vi "parse_channel_list.vi"(8 "error in (no error)":errorcluster, 11 "Channels Control":string[][](table)=[["camera", "1", "1", "", "", "", "", "", "", "", "", "", "", "", "", "", "", "", "", ""], ["probe", "1", "0", "", "", "", "", "", "", "", "", "", "", "", "", "", "", "", "", ""], ["", "1", "0", "", "", "", "", "", "", "", "", "", "", "", "", "", "", "", "", ""], ["switch 1 MOT to PGC freq shift", "1", "0", "", "", "", "", "", "", "", "", "", "", "", "", "", "", "", "", ""], ["B field", "1", "0", "", "", "", "", "", "", "", "", "", "", "", "", "", "", "", "", ""], ["trigger PD", "1", "0", "", "", "", "", "", "", "", "", "", "", "", "", "", "", "", "", ""], ["rf switch 2 cooling laser on/off", "1", "0", "", "", "", "", "", "", "", "", "", "", "", "", "", "", "", "", ""], ["Bob switch", "1", "0", "", "", "", "", "", "", "", "", "", "", "", "", "", "", "", "", ""], ["switch 3 readout freq", "1", "0", "", "", "", "", "", "", "", "", "", "", "", "", "", "", "", "", ""], ["clock trigger", "1", "0", "", "", "", "", "", "", "", "", "", "", "", "", "", "", "", "", ""]]) -> (0 "error out":errorcluster, 1 "Idle State (Binary)":u32 format="%b", 2 "# active channels":u8, 3 "Active Channels (String)":string)   [LabVIEW 2013]
panel:
  out "decimal array":u8[](array[numeric])
  out "boolean array":bool[](array[boolean])
  out "Active Channels (Binary)":u32 format="%b"
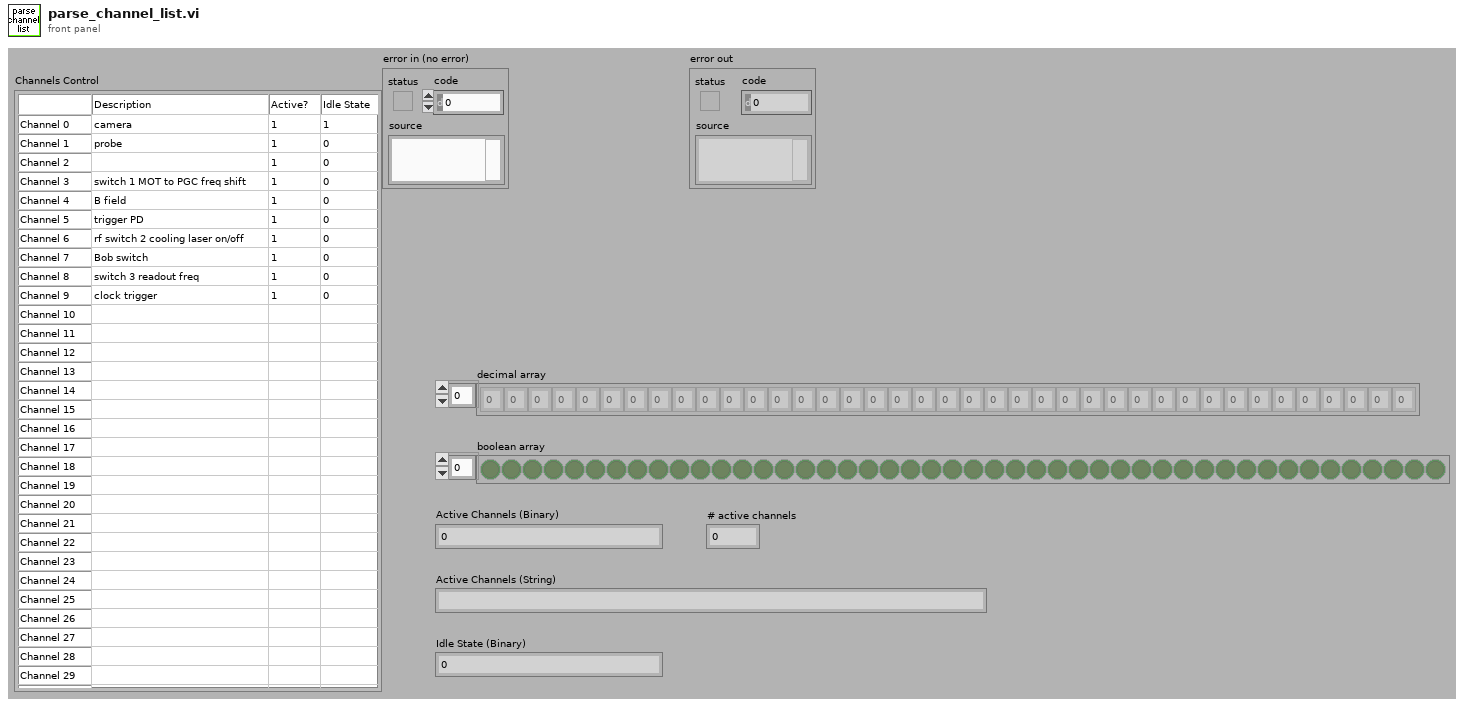
[diagram p1: front panel]
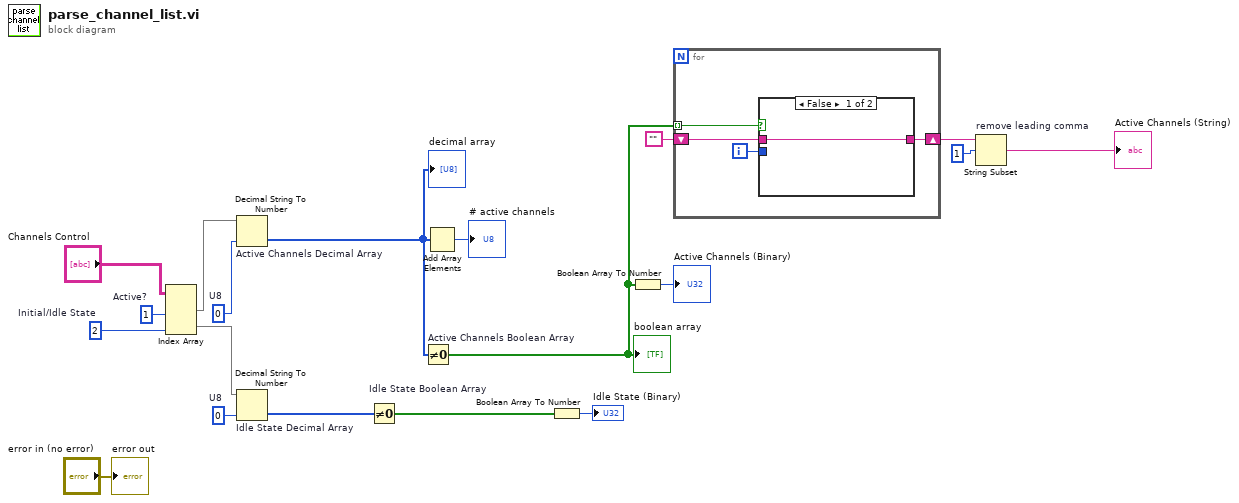
[diagram p0: block diagram]
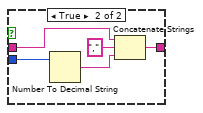
[diagram p2: hidden frame]
diagram:
  w9 = 2  # Initial/Idle State
  w11 = u8 0  # U8
  w17 = 1  # Active?
  w18 = u8 0  # U8
  n1 = Index Array(array="Channels Control", index (col) #1=w17, index (col) #2=w9) -> (element #1=w16:string[], element #2=w8:string[])  [unwired: 2 in]
  n2 = Decimal String To Number "Active Channels Decimal Array"(string=w16, default (0L)=w18) -> (number=w2:u8[])  [unwired: 1 in, 1 out]
  "decimal array" <- w2
  n3 = Decimal String To Number "Idle State Decimal Array"(string=w8, default (0L)=w11) -> (number=w10:u8[])  [unwired: 1 in, 1 out]
  n4 = Not Equal To 0? "Idle State Boolean Array"(x=w10) -> (x != 0?=w3:bool[])
  n5 = Not Equal To 0? "Active Channels Boolean Array"(x=w2) -> (x != 0?=w7:bool[])
  "boolean array" <- w7
  n6 = Add Array Elements(numeric array=w2) -> (sum=→"# active channels":u8)
  n7 = Boolean Array To Number(Boolean array=w3) -> (number=→"Idle State (Binary)":u32)
  n8 = Boolean Array To Number(Boolean array=w7) -> (number=→"Active Channels (Binary)":u32)
  n9 = for {
    tunnel: w7 -> [w20] mode=indexing
    shift-right: [w21] -> w14
    shift-left: "" -> [w23]
    i -> [w22]
    n10 = case shown="False" w20 {
      tunnel: w23 -> [w24 w29]
      tunnel: w22 -> [_ w28]
      tunnel: [w24 w27] -> w21
      frame False {
      }
      frame True {
        n11 = Number To Decimal String(number=w28) -> (decimal integer string=w26:string)  [unwired: 1 in]
        n12 = Concatenate Strings(w29, ",", w26) -> (w27:string)
      }
    }
  }
  n13 = String Subset "remove leading comma"(string=w14, offset (0)=1) -> (substring=→"Active Channels (String)":string)  [unwired: 1 in]
  "error out" <- "error in (no error)"
